vi "HEX Display To HEX ASCII.vi"(4 "Input ASCII String (HEX Display)":string) -> (1 "Output HEX ASCII (Normal Display)":string)   [LabVIEW 2011]
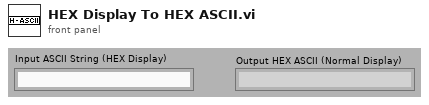
[diagram p1: front panel]
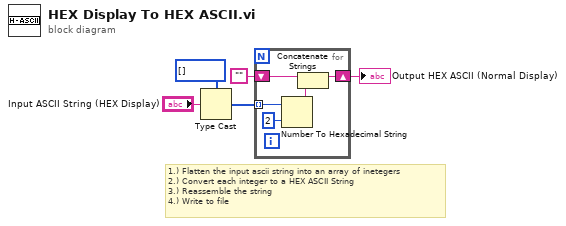
[diagram p0: block diagram]
diagram:
  # "1.) Flatten the input ascii string into an array of inetegers\n2.) Convert each integer to a HEX ASCII String\n3.) Reassemble the string\n4.) Write to file"
  n1 = Type Cast(type=u8[] [], x="Input ASCII String (HEX Display)") -> (*(type *) &x=w3:u8[])
  n2 = for {
    tunnel: w3 -> [w10] mode=indexing
    shift-right: [w6] -> w2
    shift-left: "" -> [w7]
    n3 = Number To Hexadecimal String(1:i16 2 ("width (-)"), 2:w10) -> (0:w8:string)
    n4 = Concatenate Strings(w7, w8) -> (w6:string)
  }
  "Output HEX ASCII (Normal Display)" <- w2
